vi "Write Class Data for SubPanel.vi"(8 "error in (no error)":errorcluster, 10 "Class Data for SubPanel":T1, 11 "CIF_UI in":refnum<class "CIF_UI.lvclass">) -> (0 "error out":errorcluster, 3 "CIF_UI out":refnum<class "CIF_UI.lvclass">)   [LabVIEW 2021, in "CIF_UI.lvclass"]
uses:
  CIF_UI.lvclass
  Typedef/Class Data for SubPanel.ctl
  <vilib>/gRPC/LabVIEW gRPC Library/Shared/grpcId.ctl
  Typedef/Core UI References.ctl
  Typedef/Channel Connection.ctl
  Typedef/New Plugin.ctl
  Typedef/Run Listen Button.ctl
  Typedef/CIF_Manager_UI_Tab.ctl
  Typedef/SubPanel Events.ctl
  Typedef/New Connection Event Data.ctl
  Typedef/New Connection Plugin Event Data.ctl
  CIF_UI.lvclass/CIF_UI.ctl
  <vilib>/gRPC/LabVIEW gRPC Library/grpc-lvsupport-release.lvlib
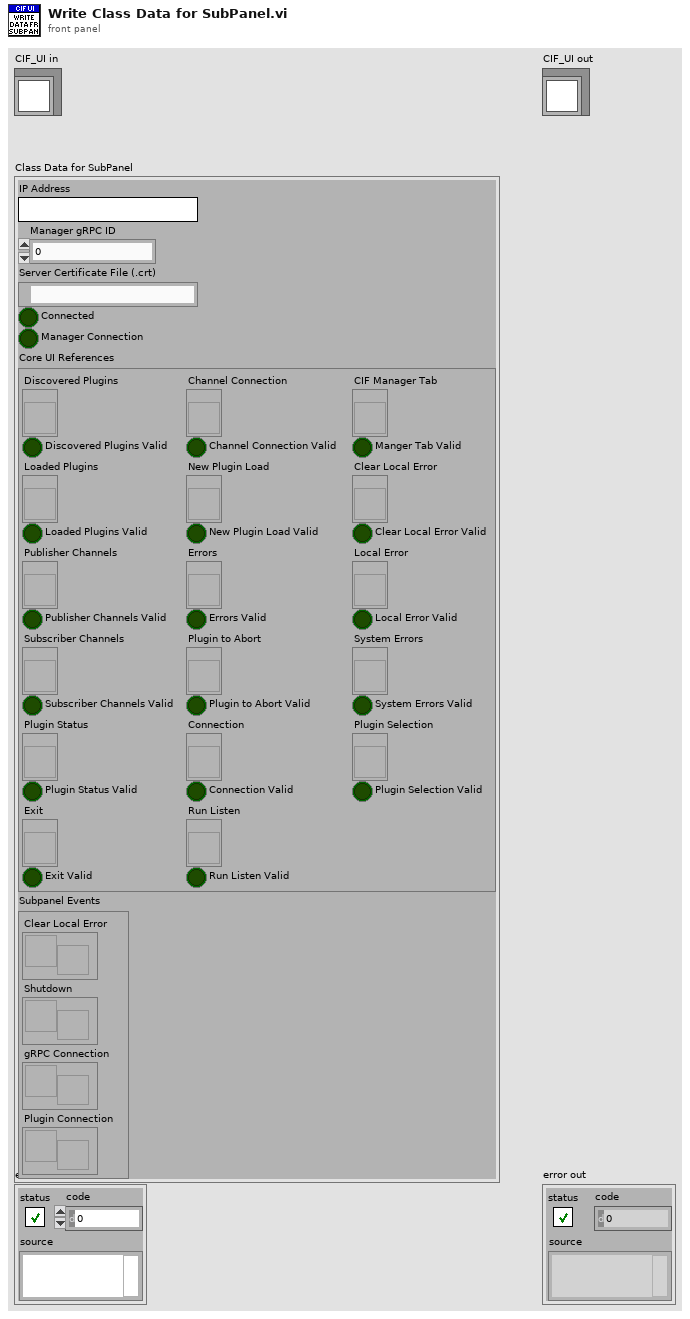
[diagram p1: front panel]
types:
  T1 = typedef "CIF_UI.lvclass/Class Data for SubPanel.ctl" = cluster{"IP Address":string, "Manager gRPC ID":T2, "Server Certificate File (.crt)":path, "Connected":bool, "Manager Connection":bool, "Core UI References":T3, "Subpanel Events":T4}
  T2 = typedef "grpc-lvsupport-release.lvlib/grpcId.ctl" = u64
  T3 = typedef "CIF_UI.lvclass/Core UI References.ctl" = cluster{"Discovered Plugins":refnum<vi>, "Discovered Plugins Valid":bool, "Loaded Plugins":refnum<vi>, "Loaded Plugins Valid":bool, "Publisher Channels":refnum<vi>, "Publisher Channels Valid":bool, "Subscriber Channels":refnum<vi>, "Subscriber Channels Valid":bool, "Plugin Status":refnum<vi>, "Plugin Status Valid":bool, "Channel Connection":refnum<vi>, "Channel Connection Valid":bool, "New Plugin Load":refnum<vi>, "New Plugin Load Valid":bool, "Errors":refnum<vi>, "Errors Valid":bool, "Plugin to Abort":refnum<vi>, "Plugin to Abort Valid":bool, "Connection":refnum<vi>, "Connection Valid":bool, "Exit":refnum<vi>, "Exit Valid":bool, "Run Listen":refnum<vi>, "Run Listen Valid":bool, "CIF Manager Tab":refnum<vi>, "Manger Tab Valid":bool, "Clear Local Error":refnum<vi>, "Clear Local Error Valid":bool, "Local Error":refnum<vi>, "Local Error Valid":bool, "System Errors":refnum<vi>, "System Errors Valid":bool, "Plugin Selection":refnum<vi>, "Plugin Selection Valid":bool}
  T4 = typedef "CIF_UI.lvclass/SubPanel Events.ctl" = cluster{"Clear Local Error":refnum<user-event>, "Shutdown":refnum<user-event>, "gRPC Connection":refnum<user-event>, "Plugin Connection":refnum<user-event>}
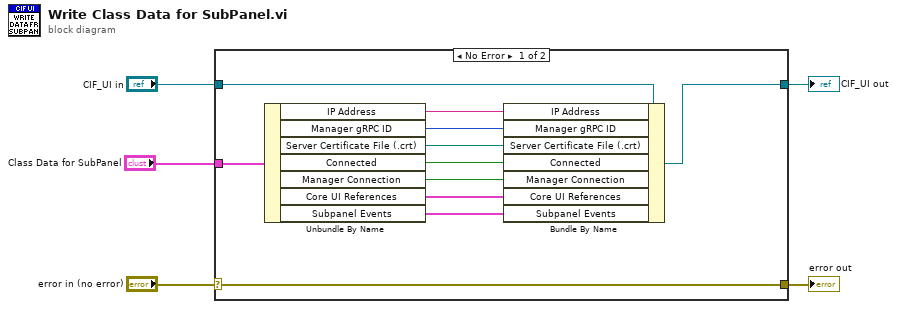
[diagram p0: block diagram]
diagram:
  n1 = case shown="No Error" "error in (no error)" {
    selector: "error in (no error)" -> [w16 w17]
    tunnel: [w16 w17] -> w4
    tunnel: [w14 w18] -> w2
    tunnel: "CIF_UI in" -> [w15 w18]
    tunnel: "Class Data for SubPanel" -> [w13 _]
    frame No Error {
      n2 = Unbundle By Name(w13) -> ("IP Address"=w12:string, "Manager gRPC ID"=w11:T2, "Server Certificate File (.crt)"=w10:path, "Connected"=w9:bool, "Manager Connection"=w8:bool, "Core UI References"=w7:T3, "Subpanel Events"=w6:T4)
      n3 = Bundle By Name(cluster=w15, "IP Address"=w12, "Manager gRPC ID"=w11, "Server Certificate File (.crt)"=w10, "Connected"=w9, "Manager Connection"=w8, "Core UI References"=w7, "Subpanel Events"=w6) -> (w14:refnum<class "CIF_UI.lvclass">)
    }
    frame Error {
    }
  }
  "error out" <- w4
  "CIF_UI out" <- w2
